vi "ReadTraitGUID.vi"(0 "Interface In":refnum<class>, 5 "error in (no error)":errorcluster) -> (14 "Interface Out":refnum<class>, 15 "GUID":string, 19 "error out":errorcluster)   [LabVIEW 2020, in "GUID Trait.lvclass"]
uses:
  GUID Trait.lvclass
panel:
  # "Place Indicators here, and remember\nto connect them to the connector pane"
  # "Place Controls here, and remember\nto connect them to the connector pane"
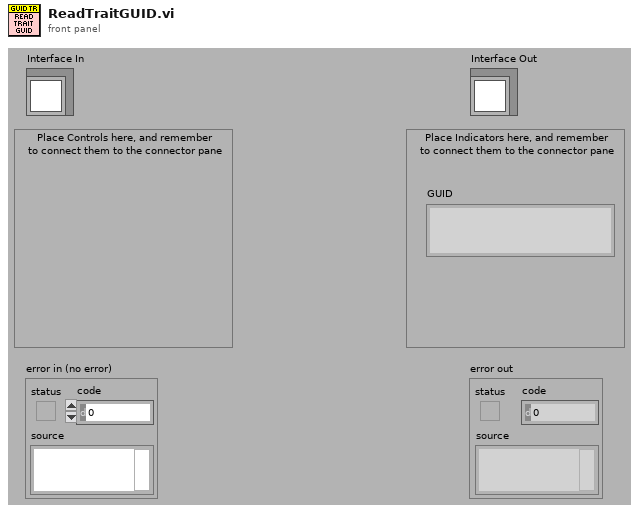
[diagram p1: front panel]
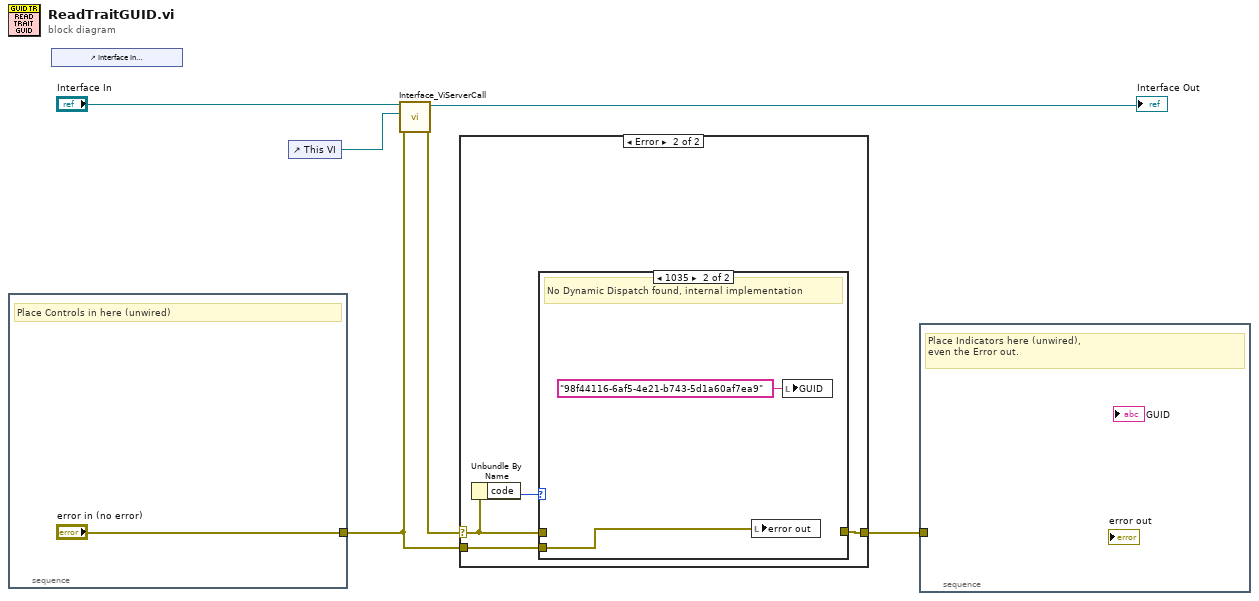
[diagram p0: block diagram]
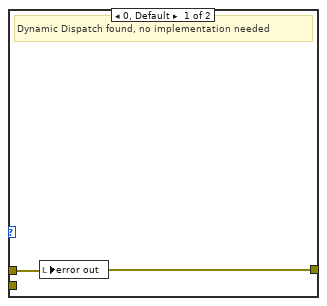
[diagram p3: hidden frame]
diagram:
  n1 = stacked-sequence {
    tunnel: ["error in (no error)"] -> w1
    frame #0 {
      # "Place Controls in here (unwired)"
    }
  }
  n2 = control-ref of="Interface In\nThis reference is needed to make sure this VI's front\npanel isn't removed when building an executable."() -> ()  [unwired: 1 out]
  n3 = control-ref of="This VI"() -> (w4:refnum<vi>)
  n4 = call <vilib>:"Interface_ViServerCall.vi"("error in (no error)"=w1, "Caller VI ref (This is the interface VI's reference)"=w4, "Interface In"="Interface In") -> ("error out"=w3:errorcluster, "Interface Out"=→"Interface Out":refnum<class>)  [unwired: 7 in]
  n5 = case shown="Error" w3 {
    selector: w3 -> [w8 w12]
    tunnel: [w8 w10] -> w2
    tunnel: w1 -> [_ w9]
    frame No Error {
    }
    frame Error {
      n6 = Unbundle By Name(w12) -> ("code"=w11:i32)
      n7 = case shown="1035" w11 {
        tunnel: w12 -> [w13 _]
        tunnel: [w13 _] -> w10
        tunnel: w9 -> [_ w15]
        frame 0, Default {
          # "Dynamic Dispatch found, no implementation needed"
          n8 = local write "error out"(w13) -> ()
        }
        frame 1035 {
          # "No Dynamic Dispatch found, internal implementation"
          n9 = local write "error out"(w15) -> ()
          n10 = local write "GUID"("98f44116-6af5-4e21-b743-5d1a60af7ea9" ("GUID")) -> ()
        }
      }
    }
  }
  n11 = stacked-sequence {
    tunnel: w2 -> [_]
    frame #0 {
      # "Place Indicators here (unwired),\neven the Error out."
    }
  }
